vi "__Set Variant Attributes with TD Validation.vi"(8 "error in (no error)":errorcluster, 9 "data":variant, 10 "String":string, 11 "Map":variant) -> (0 "error out":errorcluster, 3 "Map":variant)   [LabVIEW 2019]
uses:
  <userlib>/_OpenG.lib/lvdata/lvdata.llb/Get TDEnum from Data__ogtk.vi
  <userlib>/_OpenG.lib/lvdata/lvdata.llb/Get Data Name__ogtk.vi
  <userlib>/NEVSTOP-Programming-Palette/Configuration/ClusterCfgTable/Indexed String To Enum_nevstop.vi
  <userlib>/_OpenG.lib/error/error.llb/Build Error Cluster__ogtk.vi
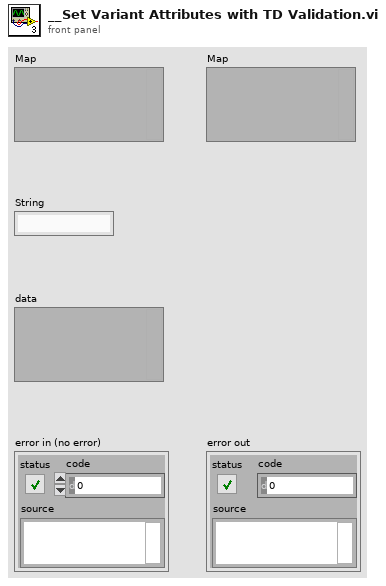
[diagram p1: front panel]
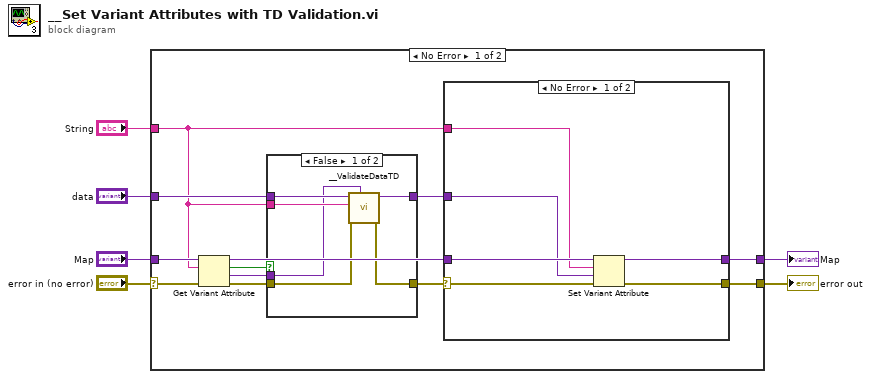
[diagram p0: block diagram]
diagram:
  n1 = case shown="No Error" "error in (no error)" {
    selector: "error in (no error)" -> [w14 w36]
    tunnel: "Map" -> [w18 w35]
    tunnel: [w17 w36] -> w5
    tunnel: [w16 w35] -> w4
    tunnel: "data" -> [w12 _]
    tunnel: "String" -> [w10 _]
    frame No Error {
      n2 = Get Variant Attribute(Variant=w18, name=w10, error in=w14) -> (duplicate Variant=w15:variant, found=w7:bool, value=w13:variant, error out=w9:errorcluster)  [unwired: 1 in]
      n3 = case shown="False" w7 {
        tunnel: w13 -> [w19 _]
        tunnel: w12 -> [w24 w26]
        tunnel: [w23 w26] -> w11
        tunnel: w10 -> [w22 _]
        tunnel: w9 -> [w21 w25]
        tunnel: [w20 w25] -> w8
        frame False {
          n4 = call "__ValidateDataTD.vi"("Expected Data"=w19, "error in (no error)"=w21, "name(\"\" as default, use data name)"=w22, "Data"=w24) -> ("error out"=w20:errorcluster, "Data out"=w23:variant)  [unwired: 6 in]
        }
        frame True {
        }
      }
      n5 = case shown="No Error" w8 {
        selector: w8 -> [w27 w34]
        tunnel: [w32 w34] -> w17
        tunnel: [w31 w33] -> w16
        tunnel: w15 -> [w30 w33]
        tunnel: w11 -> [w29 _]
        tunnel: w10 -> [w28 _]
        frame No Error {
          n6 = Set Variant Attribute(Variant=w30, name=w28, value=w29, error in=w27) -> (Variant out=w31:variant, error out=w32:errorcluster)  [unwired: 1 out]
        }
        frame Error {
        }
      }
    }
    frame Error {
    }
  }
  "error out" <- w5
  "Map" <- w4
